vi "PID Motor C1.vi"(6 "PID gains":T3={"proportional gain (Kc)"=0.05, "integral time (Ti, min)"=0.003, "derivative time (Td, min)"=0.0} {"derivative time (Td, min)" format="%.6f"; "integral time (Ti, min)" format="%.6f"; "proportional gain (Kc)" format="%.6f"}, 8 "error in (no error)":errorcluster, 9 "input":dbl, 10 "Action":T1, 11 "Setpoint C1":dbl(slide)=-0.016713091922005565 scale=-2.0..2.0) -> (0 "error out":errorcluster, 1 "dx/dt":dbl, 2 "output":dbl format="%.2f", 3 "Speed C1":T2(graph), 4 "dt out (s)":dbl format="%.3f", 5 "Counter C1":i32)   [LabVIEW 2017]
uses:
  <vilib>/myRIO/Express VI/Onboard IO/PWM/PWM Express VI.xnode
  <vilib>/addons/control/pid/NI_PID_pid.lvlib
  <vilib>/addons/control/pid/pid.llb/PID (DBL).vi
  <vilib>/myRIO/Instrument Drivers/Onboard IO/PWM/vis/Set Duty Cycle and Frequency.vi
  <vilib>/myRIO/Instrument Drivers/Onboard IO/PWM/PWM.lvlib
  <vilib>/myRIO/Instrument Drivers/Onboard IO/PWM/typedefs/PWM Configuration.ctl
  <vilib>/myRIO/Common/Instrument Driver Framework/myRIO v1.0/PWM/typedefs/PWM Channels Enum.ctl
  <vilib>/myRIO/Common/Instrument Driver Framework/Utilities/typedefs/Generic FPGA Reference.ctl
  <vilib>/myRIO/Common/Instrument Driver Framework/Utilities/typedefs/myRIO v1.0 Reference.ctl
  <vilib>/myRIO/Common/Instrument Driver Framework/Utilities/typedefs/Hardware Version Enum.ctl
  <vilib>/myRIO/Common/Instrument Driver Framework/Utilities/typedefs/myRIO Generic Hardware Reference.ctl
  <vilib>/myRIO/Instrument Drivers/Onboard IO/PWM/typedefs/PWM Reference.ctl
  <vilib>/myRIO/Instrument Drivers/Onboard IO/PWM/vis/myRIO PWM Open.xnode
  <vilib>/myRIO/Common/Instrument Driver Framework/Utilities/vis/Is FPGA Ref Available.vi
  <vilib>/myRIO/Common/Instrument Driver Framework/myRIO v1.0/PWM/vis/myRIO v1.1 Open PWM.vi
  <vilib>/userdefined/High Color/nirio_resource_hc.ctl
  enc based vel calc FGVs/Action Items.ctl
panel:
  in  "reinitialize? (F)":bool
  # "VI Description: Converts the input into a PWM value to move the motor, measures the velocity of a motor,\nthen recalculates the new input (in the form of the output)"
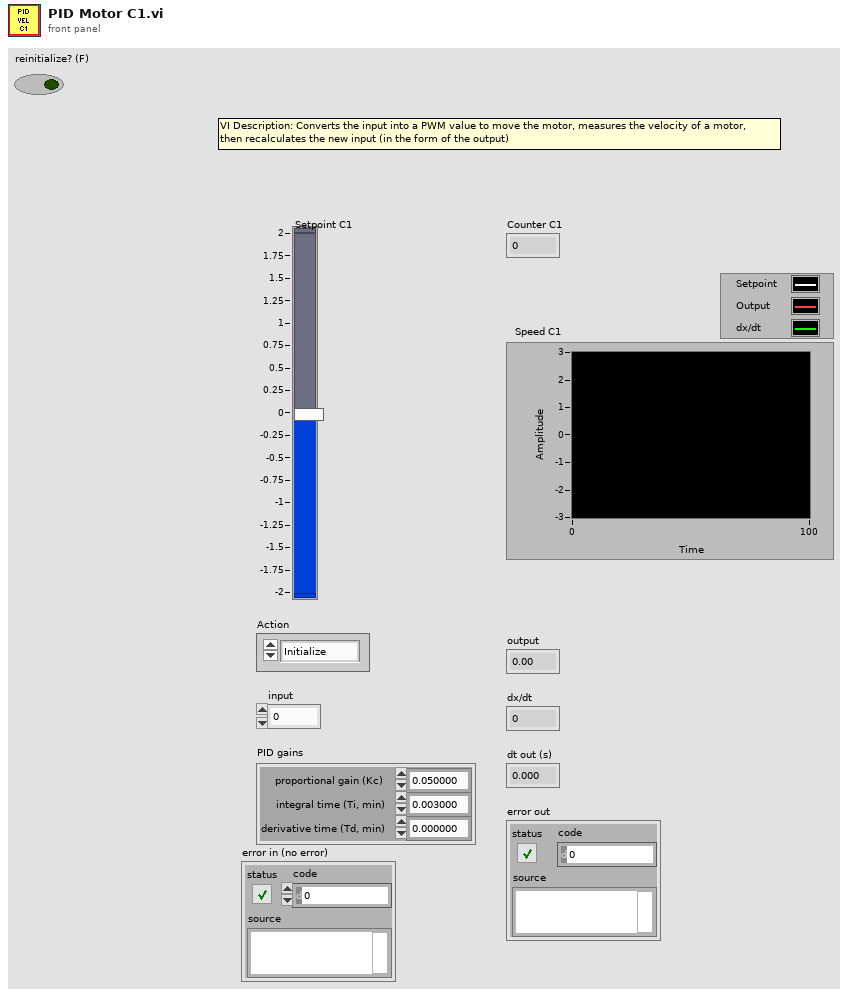
[diagram p1: front panel]
types:
  T1 = typedef "Action Items.ctl" = enum16{"Initialize", "Read"}
  T2 = cluster{"Setpoint":dbl, "output":dbl, "dx/dt":dbl}
  T3 = cluster{"proportional gain (Kc)":dbl, "integral time (Ti, min)":dbl, "derivative time (Td, min)":dbl}
  T4 = cluster{"Setpoint C1":dbl, "output":dbl, "dx/dt":dbl}
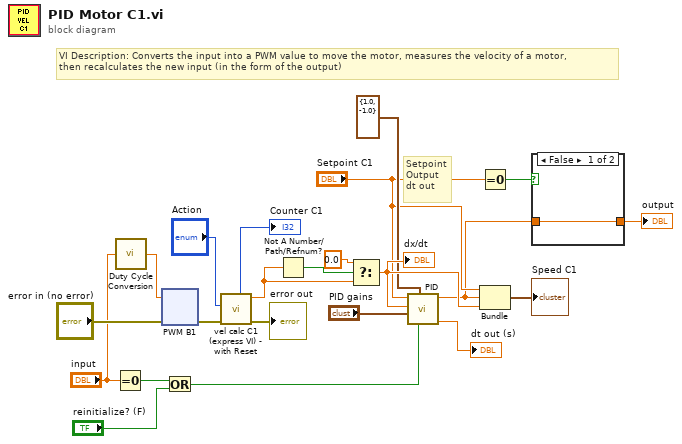
[diagram p0: block diagram]
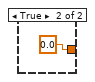
[diagram p2: hidden frame]
diagram:
  # "VI Description: Converts the input into a PWM value to move the motor, measures the velocity of a motor,\nthen recalculates the new input (in the form of the output)"
  # "Setpoint\nOutput\ndt out"
  n1 = Equal To 0?(x="input") -> (x = 0?=w3:bool)
  n2 = call "Duty Cycle Conversion.vi"("Duty Cycle In"="input") -> ("Duty Cyle Out"=w13:dbl)
  n3 = xnode "PWM B1"("error in (no error)"="error in (no error)", "Duty Cycle"=w13) -> ("error out"=w12:errorcluster)
  n4 = Or(x=w3, y="reinitialize? (F)") -> (x .or. y?=w1:bool)
  n5 = call "vel calc C1 (express VI) - with Reset.vi"("error in"=w12, "Action"="Action") -> ("error out"=→"error out":errorcluster, "dx/dt"=w21:dbl, "Counter Value"=→"Counter C1":i32)  [unwired: 5 in, 2 out]
  n6 = Not A Number/Path/Refnum?(number/path/refnum=w21) -> (NaN/Path/Refnum?=w19:bool)
  n7 = Select(t=0.0, s=w19, f=w21) -> (s? t:f=w22:dbl)
  "dx/dt" <- w22
  n8 = call-poly <vilib>:"PID.vi"("reinitialize? (F)"=w1, "output range"=cluster{"output high":dbl, "output low":dbl} {"output high"=1.0, "output low"=-1.0}, "PID gains"="PID gains", "process variable"=w22, "setpoint"="Setpoint C1") -> ("dt out (s)"=→"dt out (s)":dbl, "output"=w6:dbl)  [unwired: 5 in]
  n9 = Equal To 0?(x="Setpoint C1") -> (x = 0?=w7:bool)
  n10 = Bundle("Setpoint C1"="Setpoint C1", "output"=w6, "dx/dt"=w22) -> (→"Speed C1":T4)  [unwired: 1 in]
  n11 = case shown="False" w7 {
    tunnel: w6 -> [w23 _]
    tunnel: [w23 0.0 ("output")] -> w5
    frame False {
    }
    frame True {
    }
  }
  "output" <- w5
